vi "JL_Button_Press2.vi"(0 "GEA2 Reference In":refnum<k24>, 5 "GEA Inputs":T1={"Source"=228, "Destination"=36} {"Destination" format="%.0x"; "Source" format="%.0x"}, 7 "SingleBoard?":bool=TRUE, 9 "Button":T2, 11 "Error In":errorcluster, 12 "Hold Time (s)":dbl=0.5 format="%#_13g") -> (4 "GEA2 Reference Out":refnum<k24>, 15 "Error Out":errorcluster)   [LabVIEW 2016]
uses:
  Q:/Common/DLLs/GEA3/GeaCommunication.dll
  Common/DLLs/GEA3/GeaCommunication.dll
  Type Defs/JL_Buttons.ctl
  Common/LabVIEW GEA2 Toolkit/LabVIEW_GEA2_Toolkit.lvlibp/type defs/Source_Destination.ctl
  Common/LabVIEW GEA2 Toolkit/LabVIEW_GEA2_Toolkit.lvlibp/type defs/ERD Write Data In.ctl
  Common/LabVIEW GEA2 Toolkit/LabVIEW_GEA2_Toolkit.lvlibp/type defs/Data Type.ctl
  Common/LabVIEW GEA2 Toolkit/LabVIEW_GEA2_Toolkit.lvlibp
panel:
  out "SLB?":bool
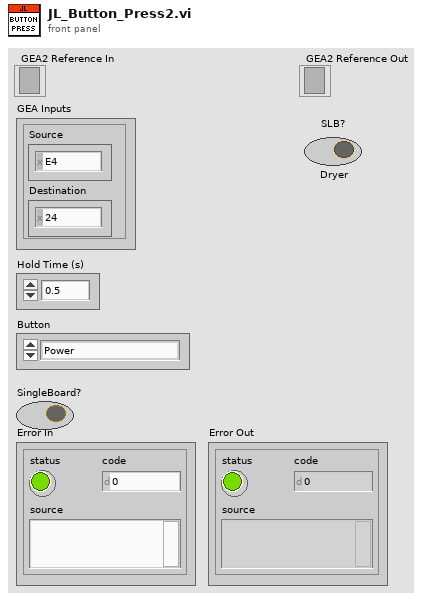
[diagram p1: front panel]
types:
  T1 = typedef "LabVIEW_GEA2_Toolkit.lvlibp/Source_Destination.ctl" = cluster{"Source":u8, "Destination":u8}
  T2 = typedef "JL_Buttons.ctl" = enum16{"Power", "Start / Pause ", "Temp Option ", "Dryness Level", "Time Option", "Time Increment ", "Time Decrement ", "MyCycle", "eDry ", "Delay", "Extended Tumble", "Control Lock", "Volume/Signal", "Damp Alert / Drum Light", "Unused", "(SW213)", "(SW322)", "Clear / Reset"}
  T3 = typedef "LabVIEW_GEA2_Toolkit.lvlibp/ERD Write Data In.ctl" = cluster{"ERD Number":u16, "Data Type":T4, "Data":string}
  T4 = typedef "LabVIEW_GEA2_Toolkit.lvlibp/Data Type.ctl" = enum16{"string", "boolean", "uint8_t", "uint16_t", "uint32_t", "uint64_t", "int8_t", "int16_t", "int32_t", "int64_t"}
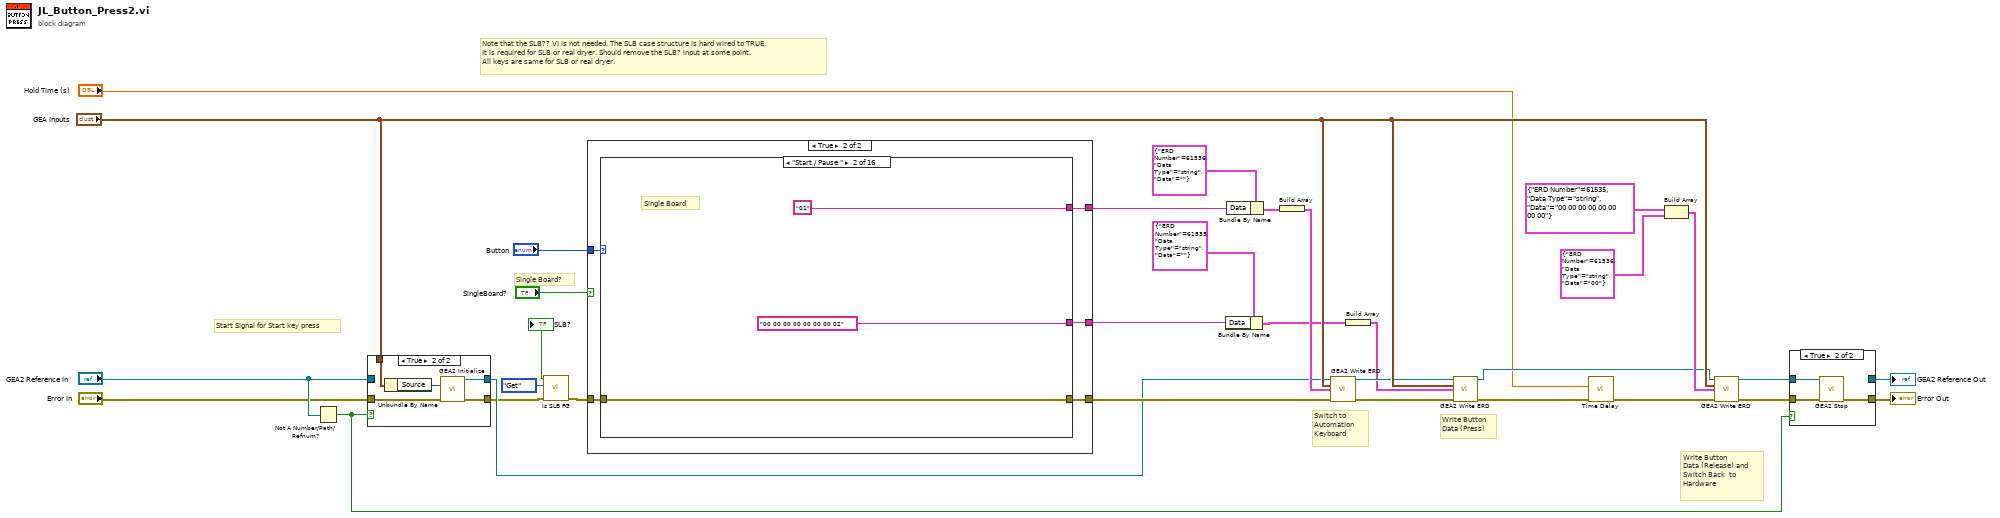
[diagram p0: block diagram]
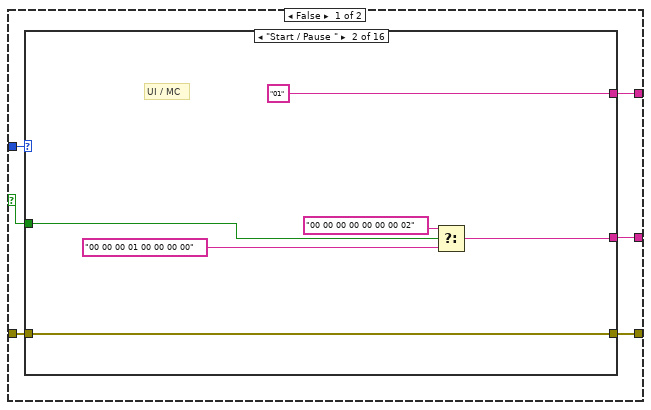
[diagram p2: hidden frame]
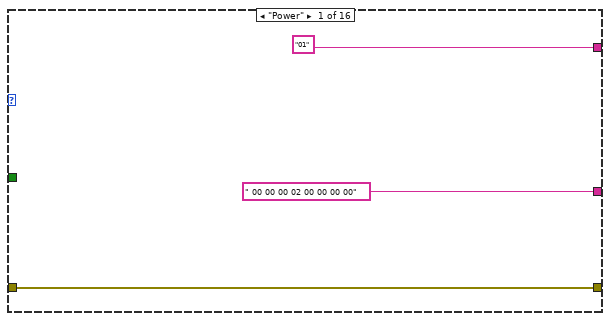
[diagram p3: hidden frame]
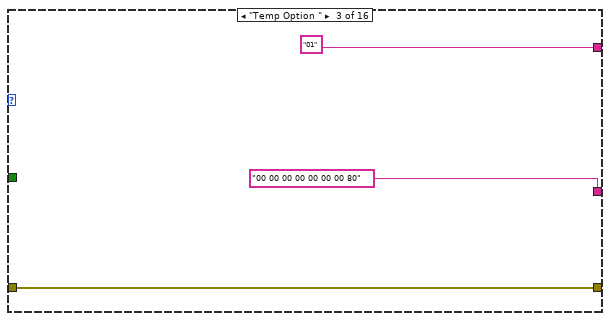
[diagram p4: hidden frame]
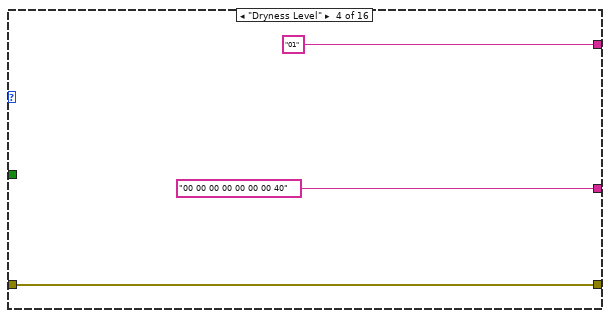
[diagram p5: hidden frame]
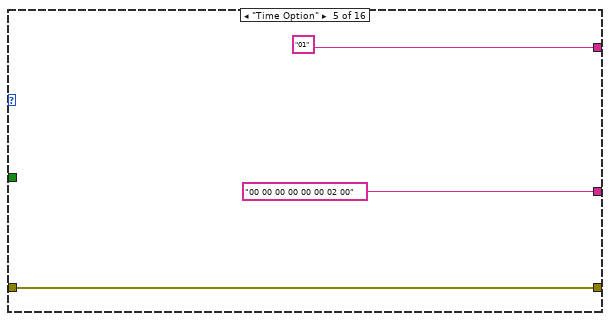
[diagram p6: hidden frame]
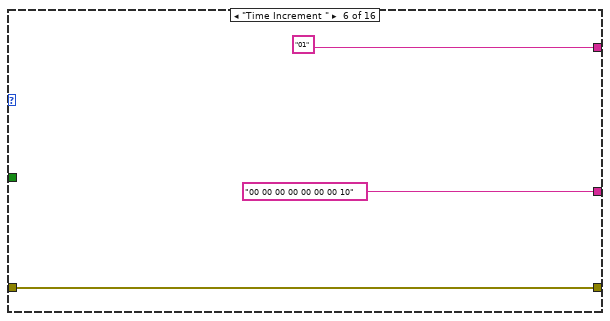
[diagram p7: hidden frame]
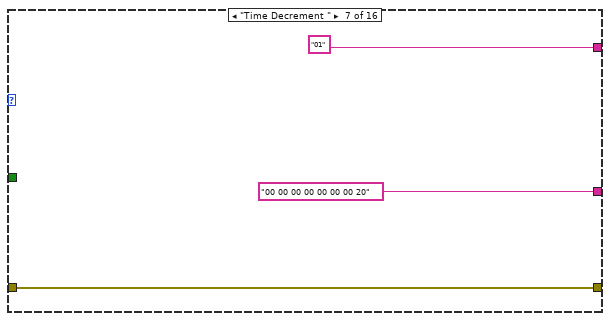
[diagram p8: hidden frame]
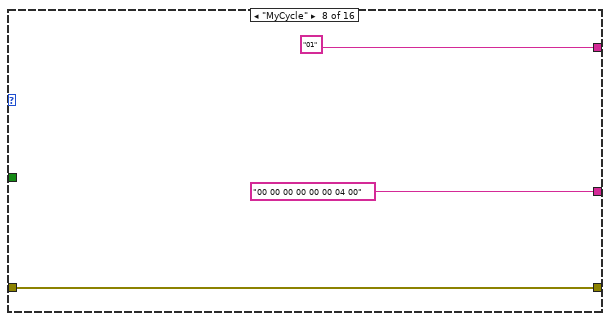
[diagram p9: hidden frame]
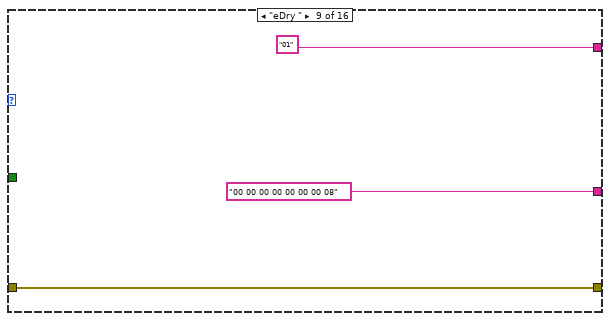
[diagram p10: hidden frame]
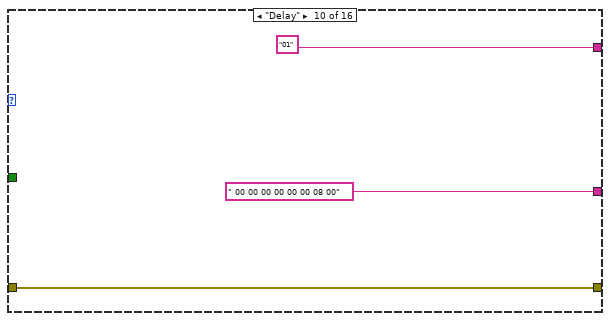
[diagram p11: hidden frame]
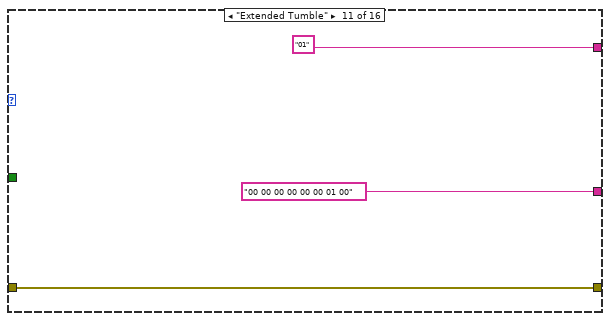
[diagram p12: hidden frame]
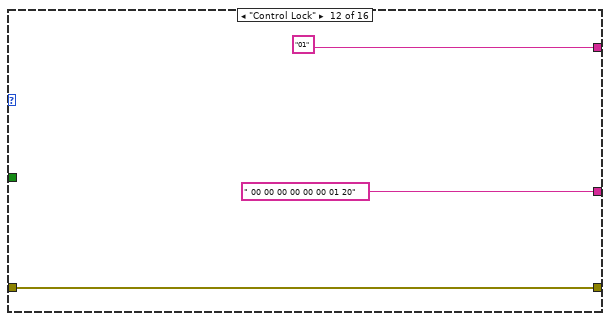
[diagram p13: hidden frame]
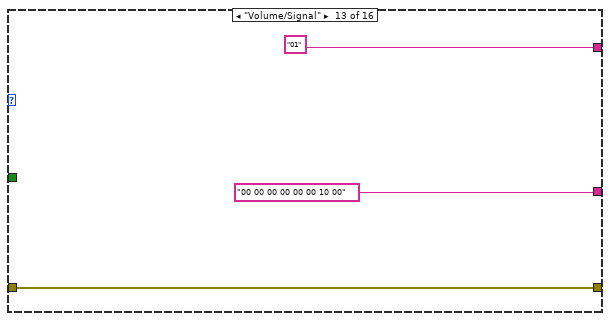
[diagram p14: hidden frame]
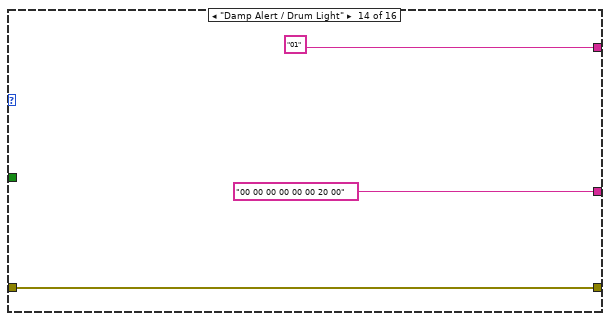
[diagram p15: hidden frame]
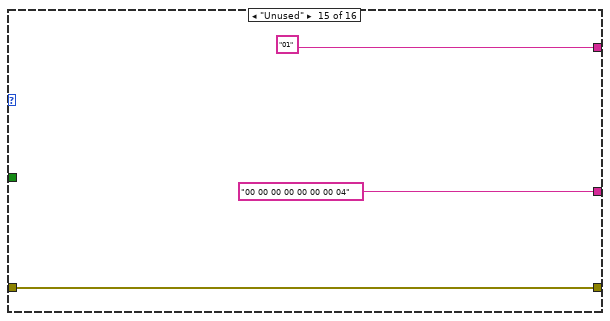
[diagram p16: hidden frame]
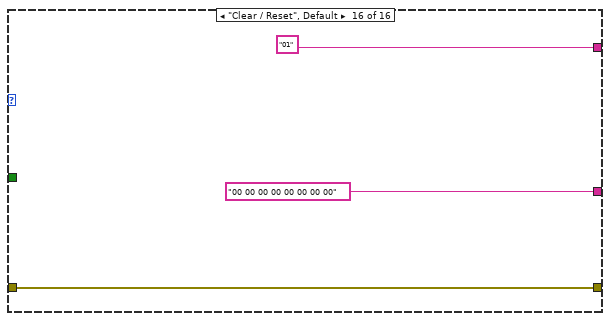
[diagram p17: hidden frame]
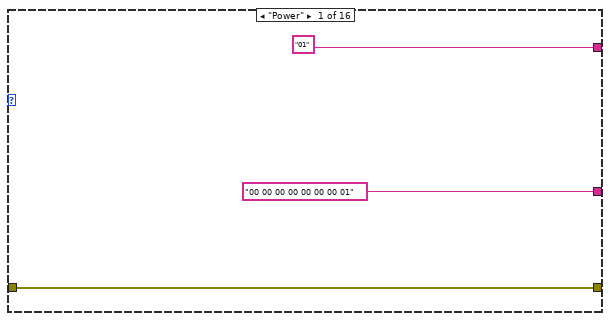
[diagram p18: hidden frame]
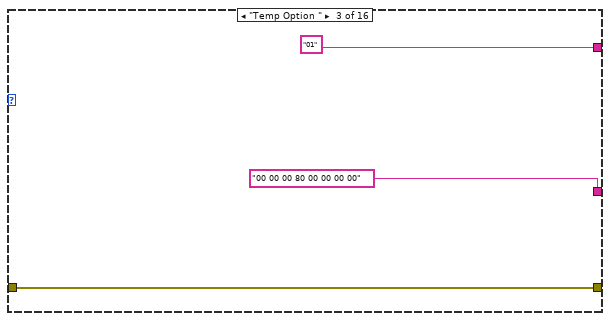
[diagram p19: hidden frame]
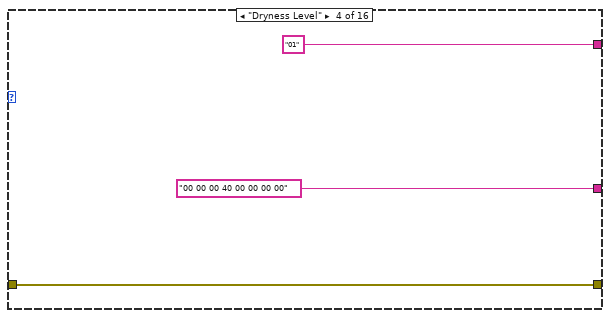
[diagram p20: hidden frame]
diagram:
  # "Note that the SLB?? VI is not needed. The SLB case structure is hard wired to TRUE.\nIt is required for SLB or real dryer. Should remove the SLB? input at some point.\nAll keys are same for SLB or real dryer."
  # "Single Board?"
  # "Start Signal for Start key press"
  # "Write Button\nData (Release) and \nSwitch Back  to\nHardware"
  # "Write Button\nData (Press)"
  # "Switch to\nAutomation \nKeyboard"
  n1 = Not A Number/Path/Refnum?(number/path/refnum="GEA2 Reference In") -> (NaN/Path/Refnum?=w30:bool)
  n2 = case shown="True" w30 {
    tunnel: "Error In" -> [w34 w40]
    tunnel: [w34 w39] -> w3
    tunnel: "GEA2 Reference In" -> [w35 _]
    tunnel: [w35 w38] -> w6
    tunnel: "GEA Inputs" -> [_ w36]
    frame False {
    }
    frame True {
      n3 = Unbundle By Name(w36) -> ("Source"=w37:u8)
      n4 = call "GEA2 Initialize.vi"("Source Address"=w37, "error in"=w40) -> ("GEA2 Reference Out"=w38:refnum<k24>, "error out"=w39:errorcluster)  [unwired: 11 in, 1 out]
    }
  }
  n5 = call "Is SLB FG.vi"("Error In"=w3, "Action"=enum16{"Get", "Set"}."Get") -> ("Error Out"=w2:errorcluster, "SLB"=→"SLB?":bool)  [unwired: 8 in]
  n6 = case shown="True" "SingleBoard?" {
    selector: "SingleBoard?" -> [w41 _]
    tunnel: [w43 w102] -> w12
    tunnel: [w44 w101] -> w11
    tunnel: w2 -> [w46 w100]
    tunnel: "Button" -> [w42 w99]
    tunnel: [w45 w98] -> w7
    frame False {
      n7 = case shown="\"Start / Pause \"" w42 {
        tunnel: ["01" "01" "01" "01" "01" "01" "01" "01" "01" "01" "01" "01" "01" "01" "01" "01"] -> w43
        tunnel: [" 00 00 00 02 00 00 00 00" w51 "00 00 00 00 00 00 00 80" "00 00 00 00 00 00 00 40" "00 00 00 00 00 00 02 00" "00 00 00 00 00 00 00 10" "00 00 00 00 00 00 00 20" "00 00 00 00 00 00 04 00" "00 00 00 00 00 00 00 08" " 00 00 00 00 00 00 08 00" "00 00 00 00 00 00 01 00" " 00 00 00 00 00 00 01 20" "00 00 00 00 00 00 10 00" "00 00 00 00 00 00 20 00" "00 00 00 00 00 00 00 04" "00 00 00 00 00 00 00 00"] -> w44
        tunnel: [w47 w50 w56 w59 w62 w65 w68 w71 w74 w77 w80 w83 w86 w89 w92 w95] -> w45
        tunnel: w46 -> [w47 w50 w56 w59 w62 w65 w68 w71 w74 w77 w80 w83 w86 w89 w92 w95]
        tunnel: w41 -> [_ w52 _ _ _ _ _ _ _ _ _ _ _ _ _ _]
        frame "Power" {
        }
        frame "Start / Pause " {
          # "UI / MC"
          n8 = Select(t="00 00 00 00 00 00 00 02", s=w52, f="00 00 00 01 00 00 00 00") -> (s? t:f=w51:string)
        }
        frame "Temp Option " {
        }
        frame "Dryness Level" {
        }
        frame "Time Option" {
        }
        frame "Time Increment " {
        }
        frame "Time Decrement " {
        }
        frame "MyCycle" {
        }
        frame "eDry " {
        }
        frame "Delay" {
        }
        frame "Extended Tumble" {
        }
        frame "Control Lock" {
        }
        frame "Volume/Signal" {
        }
        frame "Damp Alert / Drum Light" {
        }
        frame "Unused" {
        }
        frame "Clear / Reset", Default {
        }
      }
    }
    frame True {
      n9 = case shown="\"Start / Pause \"" w99 {
        tunnel: ["01" "01" "01" "01" "01" "01" "01" "01" "01" "01" "01" "01" "01" "01" "01" "01"] -> w102
        tunnel: ["00 00 00 00 00 00 00 01" "00 00 00 00 00 00 00 02" "00 00 00 80 00 00 00 00" "00 00 00 40 00 00 00 00" "00 00 02 00 00 00 00 00" "00 00 00 10 00 00 00 00" "00 00 00 20 00 00 00 00" "00 00 04 00 00 00 00 00" "00 00 00 08 00 00 00 00" "00 00 08 00 00 00 00 00" "00 00 01 00 00 00 00 00" "00 00 01 20 00 00 00 00" "00 00 10 00 00 00 00 00" "00 00 20 00 00 00 00 00" "00 00 00 00 00 00 00 04" "00 00 00 00 00 00 00 00"] -> w101
        tunnel: [w103 w106 w109 w112 w115 w118 w121 w124 w127 w130 w133 w136 w139 w142 w145 w148] -> w98
        tunnel: w100 -> [w103 w106 w109 w112 w115 w118 w121 w124 w127 w130 w133 w136 w139 w142 w145 w148]
        frame "Power" {
        }
        frame "Start / Pause " {
          # "Single Board"
        }
        frame "Temp Option " {
        }
        frame "Dryness Level" {
        }
        frame "Time Option" {
        }
        frame "Time Increment " {
        }
        frame "Time Decrement " {
        }
        frame "MyCycle" {
        }
        frame "eDry " {
        }
        frame "Delay" {
        }
        frame "Extended Tumble" {
        }
        frame "Control Lock" {
        }
        frame "Volume/Signal" {
        }
        frame "Damp Alert / Drum Light" {
        }
        frame "Unused" {
        }
        frame "Clear / Reset", Default {
        }
      }
    }
  }
  n10 = Bundle By Name(cluster=T3 {"ERD Number"=61535, "Data Type"=enum."string", "Data"=""} ("ERD Write Data In"), "Data"=w11) -> (w16:T3)
  n11 = Bundle By Name(cluster=T3 {"ERD Number"=61536, "Data Type"=enum."string", "Data"=""} ("ERD Write Data In"), "Data"=w12) -> (w27:T3)
  n12 = Build Array(w27) -> (w26:T3[])
  n13 = call "GEA2 Write ERD.vi"("GEA2 Reference In"=w6, "GEA Inputs"="GEA Inputs", "Write ERD List"=w26, "Error In"=w7) -> ("GEA2 Reference Out"=w18:refnum<k24>, "Error Out"=w21:errorcluster)  [unwired: 9 in, 1 out]
  n14 = Build Array(w16) -> (w15:T3[])
  n15 = call "GEA2 Write ERD.vi"("GEA2 Reference In"=w18, "GEA Inputs"="GEA Inputs", "Write ERD List"=w15, "Error In"=w21) -> ("GEA2 Reference Out"=w17:refnum<k24>, "Error Out"=w20:errorcluster)  [unwired: 9 in, 1 out]
  n16 = call "Time Delay"("error in (no error)"=w20, "Delay Time (s)"="Hold Time (s)") -> ("error out"=w24:errorcluster)  [unwired: 9 in]
  n17 = Build Array(T3 {"ERD Number"=61535, "Data Type"=enum."string", "Data"="00 00 00 00 00 00 00 00"} ("ERD Write Data In"), T3 {"ERD Number"=61536, "Data Type"=enum."string", "Data"="00"} ("ERD Write Data In")) -> (w25:T3[])
  n18 = call "GEA2 Write ERD.vi"("GEA2 Reference In"=w17, "GEA Inputs"="GEA Inputs", "Write ERD List"=w25, "Error In"=w24) -> ("GEA2 Reference Out"=w22:refnum<k24>, "Error Out"=w23:errorcluster)  [unwired: 9 in, 1 out]
  n19 = case shown="True" w30 {
    tunnel: [w151 w155] -> w33
    tunnel: w22 -> [w152 w154]
    tunnel: [w152 _] -> w32
    tunnel: w23 -> [w151 w153]
    frame False {
    }
    frame True {
      n20 = call "GEA2 Stop.vi"("GEA2 Reference In"=w154, "Error In"=w153) -> ("Error Out"=w155:errorcluster)  [unwired: 13 in]
    }
  }
  "Error Out" <- w33
  "GEA2 Reference Out" <- w32
